vi "read.vi"(7 "Queues":T1, 8 "error in (no error)":errorcluster, 11 "LabJackConfig":T3={"Drum Reflectors"=4, "Drum Max. Samping Window [s]"=2.0, "Drum Min. Sampling Window [s]"=0.5, "Flow Max. Samping Window [s]"=1.0, "Flow Min. Sampling Window [s]"=0.25, "Flow mL/pulse"=[1.0, 1.0, 1.0], "Flow Offset mL"=[1.0, 1.0, 1.0], "RMS Sampling Window [s]"=3.0, "TC Sampling Window [s]"=0.25, "TC Scale"=[1.0, 1.0], "TC Offset [V]"=[0.0, 0.0]} {"TC Offset [V]" format="%#_f"; "TC Scale" format="%#_f"; "Flow Offset mL" format="%#_f"; "Flow mL/pulse" format="%#_f"}) -> (0 "error out":errorcluster, 3 "Read Data":T2 {"TC [degC]" format="%#_f"; "RMS [V]" format="%#_f"; "Volume [L]" format="%#_f"; "Flow [L/min]" format="%#_f"; "Spin  [RPM]" format="%#_f"})   [LabVIEW 2025, in "LabJackEKG.lvlib"]
uses:
  LabJackEKG.lvlib
  Typedefs/LabJackData.ctl
  Typedefs/AcquisitionConfig.ctl
  Typedefs/LabJackGlobalResources.ctl
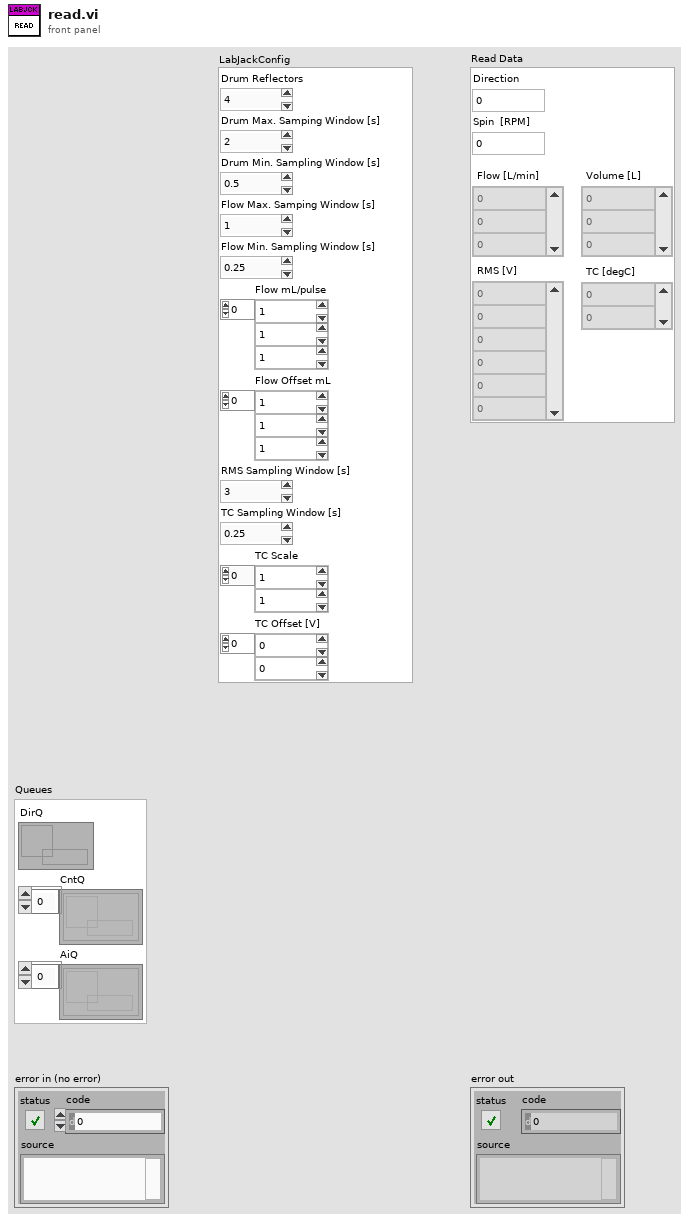
[diagram p1: front panel]
types:
  T1 = typedef "LabJackGlobalResources.ctl" = cluster{"DirQ":refnum<queue>, "CntQ":refnum<queue>[], "AiQ":refnum<queue>[]}
  T2 = typedef "LabJackEKG.lvlib/LabJackData.ctl" = cluster{"Direction":i32, "Spin  [RPM]":dbl, "Flow [L/min]":dbl[], "Volume [L]":dbl[], "RMS [V]":dbl[], "TC [degC]":dbl[]}
  T3 = typedef "LabJackEKG.lvlib/AcquisitionConfig.ctl" = cluster{"Drum Reflectors":i64, "Drum Max. Samping Window [s]":dbl, "Drum Min. Sampling Window [s]":dbl, "Flow Max. Samping Window [s]":dbl, "Flow Min. Sampling Window [s]":dbl, "Flow mL/pulse":dbl[], "Flow Offset mL":dbl[], "RMS Sampling Window [s]":dbl, "TC Sampling Window [s]":dbl, "TC Scale":dbl[], "TC Offset [V]":dbl[]}
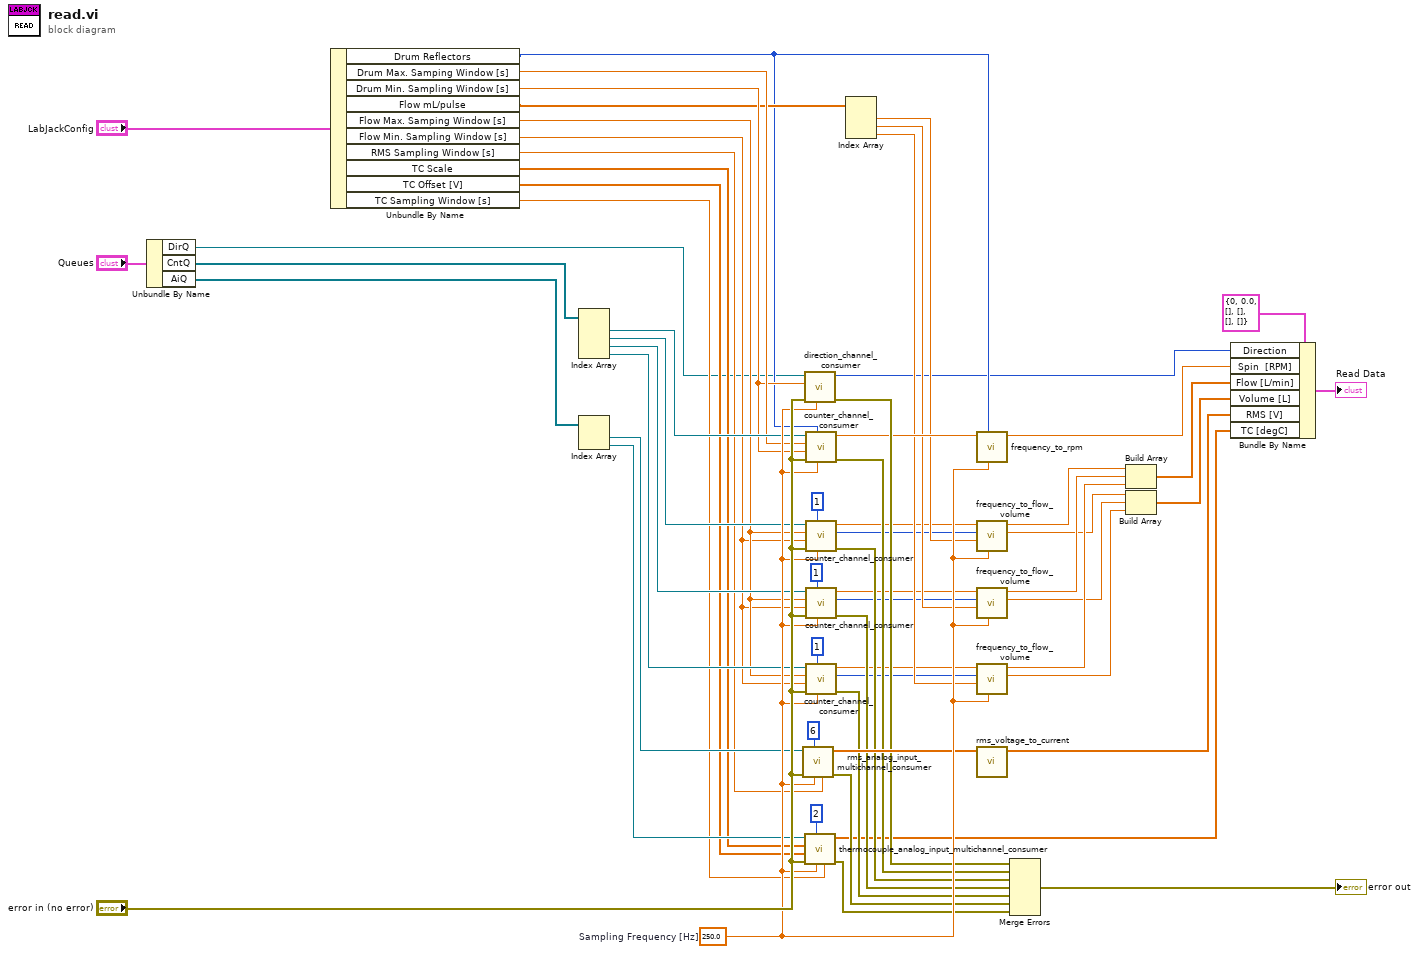
[diagram p0: block diagram]
diagram:
  w58 = 250.0  # Sampling Frequency [Hz]
  n1 = Unbundle By Name("Queues") -> ("DirQ"=w2:refnum<queue>, "CntQ"=w3:refnum<queue>[], "AiQ"=w1:refnum<queue>[])
  n2 = Unbundle By Name("LabJackConfig") -> ("Drum Reflectors"=w27:i64, "Drum Max. Samping Window [s]"=w37:dbl, "Drum Min. Sampling Window [s]"=w36:dbl, "Flow mL/pulse"=w35:dbl[], "Flow Max. Samping Window [s]"=w34:dbl, "Flow Min. Sampling Window [s]"=w33:dbl, "RMS Sampling Window [s]"=w32:dbl, "TC Scale"=w31:dbl[], "TC Offset [V]"=w30:dbl[], "TC Sampling Window [s]"=w29:dbl)
  n3 = Index Array(array=w3) -> (element #1=w56:refnum<queue>, element #2=w55:refnum<queue>, element #3=w54:refnum<queue>, element #4=w53:refnum<queue>)  [unwired: 4 in]
  n4 = Index Array(array=w1) -> (element #1=w47:refnum<queue>, element #2=w48:refnum<queue>)  [unwired: 2 in]
  n5 = call "rms_analog_input_multichannel_consumer.vi"("Sampling Window [s]"=w32, "Sampling Frequency [Hz]"=w58, "Number of Channels"=6, "error in (no error)"="error in (no error)", "queue out"=w47) -> ("error out"=w44:errorcluster, "RMS [V]"=w46:dbl[])  [unwired: 5 in]
  n6 = call "direction_channel_consumer.vi"("Sampling Frequency [Hz]"=w58, "error in (no error)"="error in (no error)", "Sampling Offset [s]"=w36, "DirQ"=w2) -> ("error out"=w39:errorcluster, "Direction"=w11:i32)  [unwired: 6 in]
  n7 = call "thermocouple_analog_input_multichannel_consumer.vi"("Sampling Window [s]"=w29, "Sampling Frequency [Hz]"=w58, "Number of Channels"=2, "error in (no error)"="error in (no error)", "Offset"=w30, "Scale"=w31, "queue out"=w48) -> ("error out"=w45:errorcluster, "TC [degC]"=w5:dbl[])  [unwired: 1 in, 2 out]
  n8 = call "counter_channel_consumer.vi"("Sampling Frequency [Hz]"=w58, "Sample Group Size"=w27, "error in (no error)"="error in (no error)", "Min. Sampling Window [s]"=w36, "Max. Samping Window [s]"=w37, "Queue in"=w56) -> ("error out"=w40:errorcluster, "Pulse Frequency [Hz]"=w28:dbl)  [unwired: 4 out]
  n9 = call "counter_channel_consumer.vi"("Sampling Frequency [Hz]"=w58, "Sample Group Size"=i64 1, "error in (no error)"="error in (no error)", "Min. Sampling Window [s]"=w33, "Max. Samping Window [s]"=w34, "Queue in"=w55) -> ("error out"=w41:errorcluster, "Pulse Count"=w20:i64, "Pulse Frequency [Hz]"=w21:dbl)  [unwired: 3 out]
  n10 = call "counter_channel_consumer.vi"("Sampling Frequency [Hz]"=w58, "Sample Group Size"=i64 1, "error in (no error)"="error in (no error)", "Min. Sampling Window [s]"=w33, "Max. Samping Window [s]"=w34, "Queue in"=w54) -> ("error out"=w42:errorcluster, "Pulse Count"=w19:i64, "Pulse Frequency [Hz]"=w23:dbl)  [unwired: 3 out]
  n11 = call "counter_channel_consumer.vi"("Sampling Frequency [Hz]"=w58, "Sample Group Size"=i64 1, "error in (no error)"="error in (no error)", "Min. Sampling Window [s]"=w33, "Max. Samping Window [s]"=w34, "Queue in"=w53) -> ("error out"=w43:errorcluster, "Pulse Count"=w18:i64, "Pulse Frequency [Hz]"=w22:dbl)  [unwired: 3 out]
  n12 = Index Array(array=w35) -> (element #1=w26:dbl, element #2=w24:dbl, element #3=w25:dbl)  [unwired: 3 in]
  n13 = call "frequency_to_rpm.vi"("Sampling Frequency [Hz]"=w58, "Number of Stickers"=w27, "Pulse Frequency [Hz]"=w28) -> ("Spin [RPM]"=w9:dbl)  [unwired: 8 in]
  n14 = call "frequency_to_flow_volume.vi"("Sampling Frequency [Hz]"=w58, "mlL/pulse"=w26, "Pulse Count"=w20, "Pulse Frequency [Hz]"=w21) -> ("Volume [L]"=w14:dbl, "Flow [L/min]"=w17:dbl)  [unwired: 6 in]
  n15 = call "frequency_to_flow_volume.vi"("Sampling Frequency [Hz]"=w58, "mlL/pulse"=w24, "Pulse Count"=w19, "Pulse Frequency [Hz]"=w23) -> ("Volume [L]"=w13:dbl, "Flow [L/min]"=w16:dbl)  [unwired: 6 in]
  n16 = call "frequency_to_flow_volume.vi"("Sampling Frequency [Hz]"=w58, "mlL/pulse"=w25, "Pulse Count"=w18, "Pulse Frequency [Hz]"=w22) -> ("Volume [L]"=w12:dbl, "Flow [L/min]"=w15:dbl)  [unwired: 6 in]
  n17 = call "rms_voltage_to_current.vi"("RMS [V]"=w46) -> ("RMS[A]"=w6:dbl[])  [unwired: 10 in]
  n18 = Merge Errors(w39, w40, w41, w42, w43, w44, w45) -> (→"error out":errorcluster)
  n19 = Build Array(w17, w16, w15) -> (w8:dbl[])
  n20 = Build Array(w14, w13, w12) -> (w7:dbl[])
  n21 = Bundle By Name(cluster=T2 {"Direction"=0, "Spin  [RPM]"=0.0, "Flow [L/min]"=[], "Volume [L]"=[], "RMS [V]"=[], "TC [degC]"=[]} ("LabJack Data"), "Direction"=w11, "Spin  [RPM]"=w9, "Flow [L/min]"=w8, "Volume [L]"=w7, "RMS [V]"=w6, "TC [degC]"=w5) -> (→"Read Data":T2)
